vi "XYZStage-Move command.vi"(8 "Error In":errorcluster, 9 "XYZ Stage data":T2={"Command"=enum."Initialize", "Channel"="Z", "X"=0.0, "Y"=0.0, "Z"=0.0, "Speed"=0, "Zero"=FALSE, "Use acknowledgement?"=TRUE} {"Speed" format="Speed= %.0f"; "Z" format="Z= %#_g"; "Y" format="Y= %#_g"; "X" format="X= %#_g"}, 10 "Z Stage":T1, 11 "XYZ Stage config":T5={"COM port"="COM7", "Baudrate"=0, "Type"=""}) -> (0 "Error Out":errorcluster, 1 "Move XYZ command String":string)   [LabVIEW 2020]
uses:
  Typedefs/XY Stage config cluster.ctl
  Typedefs/XYZ stage data.ctl
  Typedefs/XYZ stage states.ctl
  Typedefs/XYZ channel ring.ctl
  Typedefs/Z Stage config cluster.ctl
  Typedefs/Z intelock check type.ctl
  Global Variables/General Globals.vi
panel:
  out "Current Pos":dbl format="%#.3f"
  in  "Absolute (0.0 um)":dbl format="%.1f"
  in  "Step (0.0 um)":dbl format="%.1f"
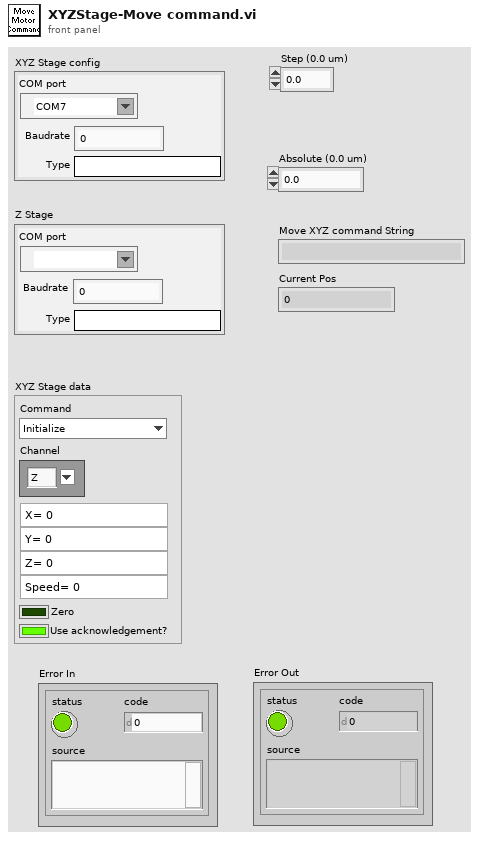
[diagram p1: front panel]
types:
  T1 = typedef "Z Stage config cluster.ctl" = cluster{"COM port":refnum<visa-resource-name>, "Baudrate":i32, "Type":string}
  T2 = typedef "XYZ stage data.ctl" = cluster{"Command":T3, "Channel":T4, "X":sgl, "Y":sgl, "Z":sgl, "Speed":i32, "Zero":bool, "Use acknowledgement?":bool}
  T3 = typedef "XYZ stage states.ctl" = enum16{"Dequeue", "Initialize", "Read Position", "Read Speed Setting", "Move", "Set Max Speed", "Reset Axis", "Stop all movement"}
  T4 = typedef "XYZ channel ring.ctl" = string
  T5 = typedef "XY Stage config cluster.ctl" = cluster{"COM port":refnum<visa-resource-name>, "Baudrate":i32, "Type":string}
  T6 = typedef "Z intelock check type.ctl" = enum16{"Check against Z limit", "Check againt current position"}
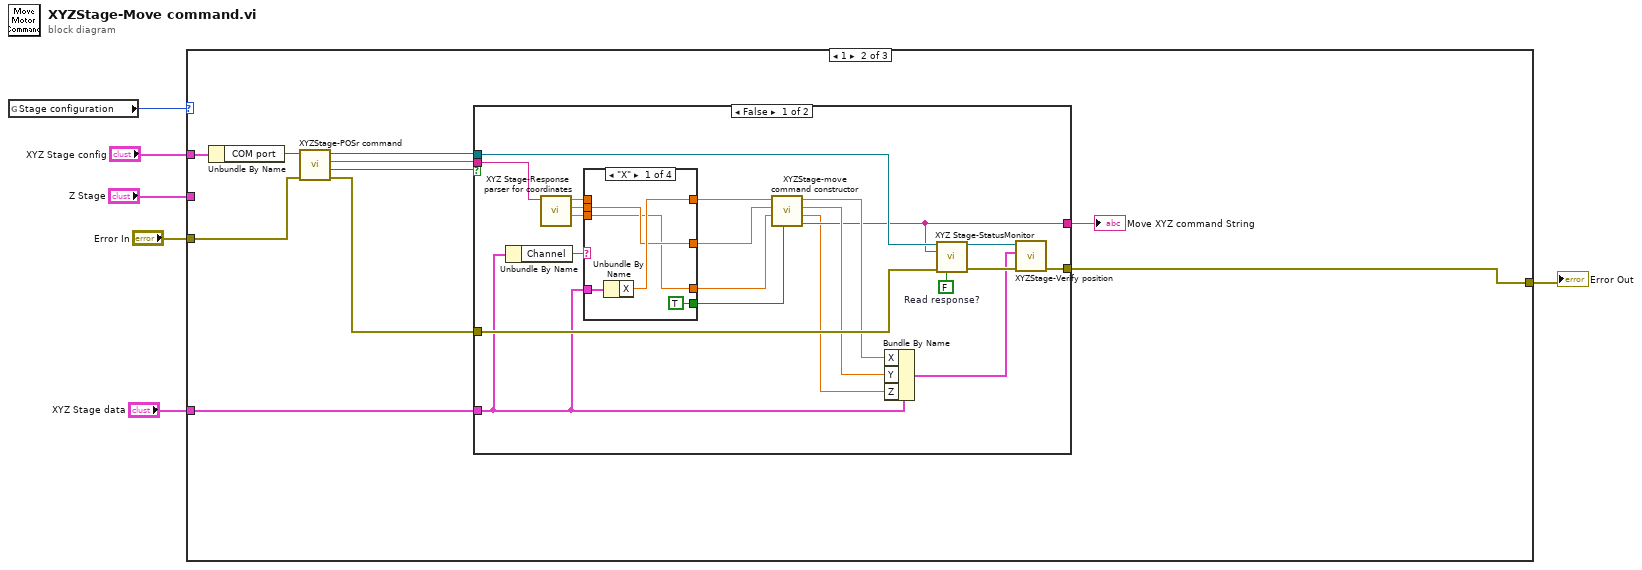
[diagram p0: block diagram]
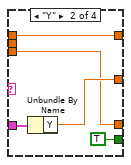
[diagram p3: hidden frame]
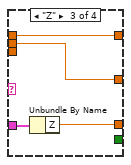
[diagram p4: hidden frame]
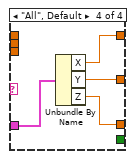
[diagram p5: hidden frame]
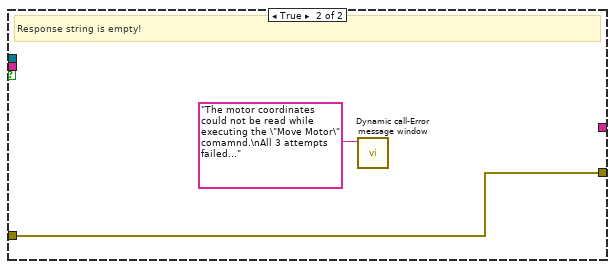
[diagram p6: hidden frame]
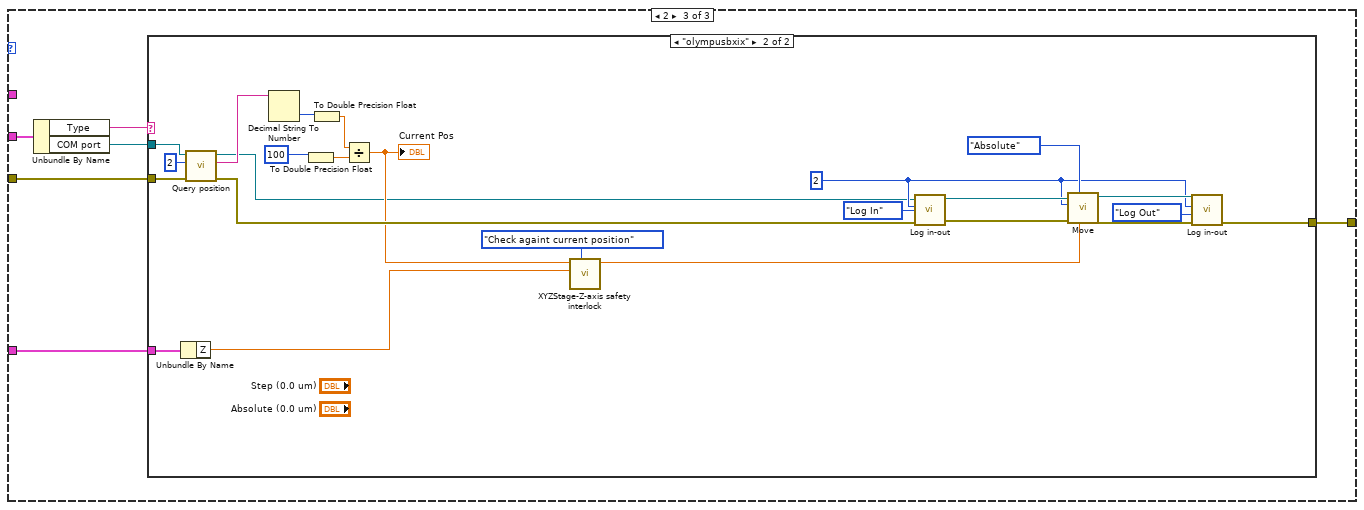
[diagram p7: hidden frame]
diagram:
  n1 = global read "General Globals.vi" "Stage configuration"() -> (w3:i32)
  n2 = case shown="1" w3 {
    tunnel: "XYZ Stage config" -> [_ w15 _]
    tunnel: "XYZ Stage data" -> [_ w13 w59]
    tunnel: "Error In" -> [w7 w10 w61]
    tunnel: "Z Stage" -> [_ _ w64]
    tunnel: [w7 w8 w60] -> w1
    frame 0, Default {
    }
    frame 1 {
      n3 = Unbundle By Name(w15) -> ("COM port"=w17:refnum<visa-resource-name>)
      n4 = call "XYZStage-POSr command.vi"("Error in"=w10, "VISA Refnum in"=w17) -> ("Error out"=w9:errorcluster, "Empty response string"=w11:bool, "read string"=w16:string, "VISA Refnum out"=w14:refnum<visa-resource-name>)  [unwired: 6 in]
      n5 = case shown="False" w11 {
        tunnel: w9 -> [w38 w58]
        tunnel: w16 -> [w37 _]
        tunnel: w14 -> [w36 _]
        tunnel: [w30 w58] -> w8
        tunnel: w13 -> [w26 _]
        tunnel: [w22 _] -> w12
        frame False {
          w28 = FALSE  # Read response?
          n6 = Unbundle By Name(w26) -> ("Channel"=w35:T4)
          n7 = call "XYZ Stage-Response parser for coordinates.vi"("Filtered response string (no CR)"=w37) -> ("Z"=w32:sgl, "Y"=w33:sgl, "X"=w34:sgl)  [unwired: 7 in, 1 out]
          n8 = case shown="\"X\"" w35 {
            tunnel: [w42 w47 w50 w56] -> w21
            tunnel: [w41 w46 w49 w55] -> w27
            tunnel: [w40 w45 w51 w54] -> w20
            tunnel: w26 -> [w43 w48 w52 w53]
            tunnel: w34 -> [_ w47 w50 _]
            tunnel: w33 -> [w41 _ w49 _]
            tunnel: w32 -> [w40 w45 _ _]
            tunnel: [TRUE TRUE _ _] -> w18
            frame "X" {
              n9 = Unbundle By Name(w43) -> ("X"=w42:sgl)
            }
            frame "Y" {
              n10 = Unbundle By Name(w48) -> ("Y"=w46:sgl)
            }
            frame "Z" {
              n11 = Unbundle By Name(w52) -> ("Z"=w51:sgl)
            }
            frame "All", Default {
              n12 = Unbundle By Name(w53) -> ("X"=w56:sgl, "Y"=w55:sgl, "Z"=w54:sgl)
            }
          }
          n13 = call "XYZStage-move command constructor.vi"("Bypass Z-safety interlock"=w18, "Z"=w20, "Y"=w27, "X"=w21) -> ("Move command"=w22:string, "Adjusted Z"=w19:sgl, "Adjusted Y"=w23:sgl, "Adjusted X"=w24:sgl)  [unwired: 3 in, 1 out]
          n14 = Bundle By Name(cluster=w26, "X"=w24, "Y"=w23, "Z"=w19) -> (w25:T2)
          n15 = call "XYZ Stage-StatusMonitor.vi"("VISA resource name"=w36, "string to write"=w22, "Error In"=w38, "Read response? (T)"=w28) -> ("VISA resource name out"=w29:refnum<visa-resource-name>, "Error Out"=w31:errorcluster)  [unwired: 7 in, 3 out]
          n16 = call "XYZStage-Verify position.vi"("error in (no error)"=w31, "XYZ Stage data"=w25, "XYZ Stage Port"=w29) -> ("error out"=w30:errorcluster)  [unwired: 8 in]
        }
        frame True {
          # "Response string is empty!"
          n17 = call "Dynamic call-Error message window.vi"("Error Message"="The motor coordinates could not be read while executing the \"Move Motor\" comamnd.\nAll 3 attempts failed...") -> ()  [unwired: 10 in, 1 out]
        }
      }
      "Move XYZ command String" <- w12
    }
    frame 2 {
      n18 = Unbundle By Name(w64) -> ("Type"=w63:string, "COM port"=w62:refnum<visa-resource-name>)
      n19 = case shown="\"olympusbxix\"" w63 {
        tunnel: w62 -> [_ w82]
        tunnel: w61 -> [w65 w83]
        tunnel: [w65 w80] -> w60
        tunnel: w59 -> [_ w68]
        frame "False", Default {
        }
        frame "olympusbxix" {
          w71 = 2 ("Device Number (1)")
          n20 = Unbundle By Name(w68) -> ("Z"=w67:sgl)
          n21 = call "Query position.vi"("error in (no error)"=w83, "Device Number (1)"=2, "VISA Resource Name"=w82) -> ("error out"=w81:errorcluster, "Result"=w89:string, "VISA Resource Name Out"=w66:refnum<visa-resource-name>)  [unwired: 6 in]
          n22 = Decimal String To Number(string=w89) -> (number=w88:i32)  [unwired: 2 in, 1 out]
          n23 = To Double Precision Float(number=100 ("y")) -> (double precision float=w87:dbl)
          n24 = To Double Precision Float(number=w88) -> (double precision float=w85:dbl)
          n25 = Divide(x=w85, y=w87) -> (x/y=w70:dbl)
          "Current Pos" <- w70
          n26 = call "XYZStage-Z-axis safety interlock.vi"("Interlock check type"=Z_intelock_check_type."Check againt current position", "Z move to"=w67, "Z Current"=w70) -> ("Z"=w79:sgl)  [unwired: 7 in, 1 out]
          n27 = call "Log in-out.vi"("error in (no error)"=w81, "Input"=enum16{"Log In", "Log Out"}."Log In", "Device Number (1)"=w71, "VISA Resource Name"=w66) -> ("error out"=w76:errorcluster, "VISA Resource Name Out"=w77:refnum<visa-resource-name>)  [unwired: 5 in, 1 out]
          n28 = call "Move.vi"("Absolute (0.0 um)"=w79, "Direction (1: Down)"=enum16{"Up", "Down", "Absolute"}."Absolute", "error in (no error)"=w76, "Device Number (1)"=w71, "VISA Resource Name"=w77) -> ("error out"=w75:errorcluster, "VISA Resource Name Out"=w72:refnum<visa-resource-name>)  [unwired: 4 in, 1 out]
          n29 = call "Log in-out.vi"("error in (no error)"=w75, "Input"=enum16{"Log In", "Log Out"}."Log Out", "Device Number (1)"=w71, "VISA Resource Name"=w72) -> ("error out"=w80:errorcluster)  [unwired: 5 in, 2 out]
        }
      }
    }
  }
  "Error Out" <- w1
